vi "Read ID.vi"(8 "error in (no error)":errorcluster, 11 "289 in":refnum<class "289.lvclass">) -> (0 "error out":errorcluster, 3 "289 out":refnum<class "289.lvclass">)   [LabVIEW 2015, in "289.lvclass"]
doc: "VI used to Read Hardware ID"
uses:
  289.lvclass
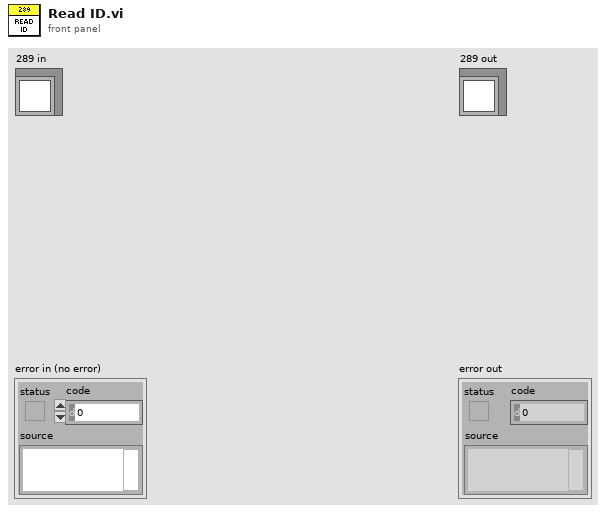
[diagram p1: front panel]
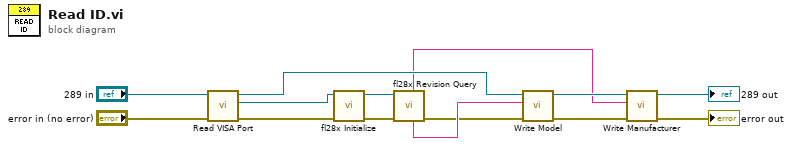
[diagram p0: block diagram]
diagram:
  n1 = call-dynamic "Read VISA Port.vi"("error in (no error)"="error in (no error)", "Device in"="289 in") -> ("error out"=w6:errorcluster, "VISA Port"=w7:refnum<visa-resource-name>, "Device out"=w10:refnum<class "289.lvclass">)  [unwired: 7 in]
  n2 = call "fl28x Initialize.vi"("error in (no error)"=w6, "VISA resource name"=w7) -> ("error out"=w5:errorcluster, "VISA resource name out"=w4:refnum<visa-resource-name>)  [unwired: 8 in]
  n3 = call "fl28x Revision Query.vi"("error in (no error)"=w5, "VISA session"=w4) -> ("error out"=w1:errorcluster, "Modelo"=w2:string, "Fabricante"=w3:string)  [unwired: 4 in, 3 out]
  n4 = call-dynamic "Write Model.vi"("error in (no error)"=w1, "Model"=w2, "Device in"=w10) -> ("error out"=w12:errorcluster, "Device out"=w9:refnum<class "289.lvclass">)  [unwired: 7 in]
  n5 = call-dynamic "Write Manufacturer.vi"("error in (no error)"=w12, "Manufacturer"=w3, "Device in"=w9) -> ("error out"=→"error out":errorcluster, "Device out"=→"289 out":refnum<class "289.lvclass">)  [unwired: 7 in]
